vi "I2C_MASTER_READ.vi"(0 "error in (no error)":errorcluster) -> (1 "Arduino Data":T1, 2 "error out":errorcluster)   [LabVIEW 2018]
uses:
  <vilib>/Studica/Studica Toolkit/Background/I2C Channel.ctl
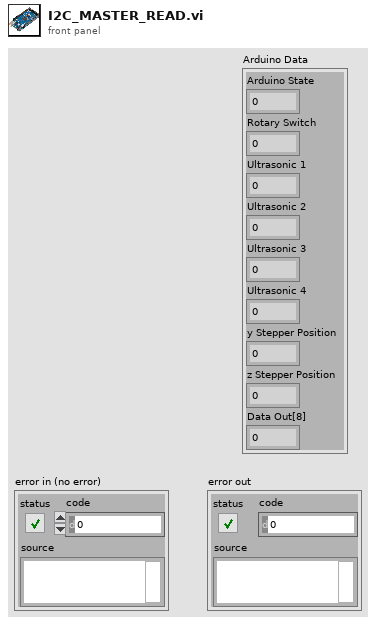
[diagram p1: front panel]
types:
  T1 = cluster{"Arduino State":u8, "Rotary Switch":u8, "Ultrasonic 1":u8, "Ultrasonic 2":u8, "Ultrasonic 3":u8, "Ultrasonic 4":u8, "y Stepper Position":u8, "z Stepper Position":u8, "Data Out[8]":u8}
  T2 = typedef "I2C Channel.ctl" = enum16{"Not Connected", "A", "B"}
  T3 = cluster{"I2C Channel":T2, "FPGA VI Reference Out":refnum<k20>}
  T4 = cluster{"Data Out[0]":u8, "Data Out[1]":u8, "Data Out[2]":u8, "Data Out[3]":u8, "Data Out[4]":u8, "Data Out[5]":u8, "Data Out[6]":u8, "Data Out[7]":u8, "Data Out[8]":u8}
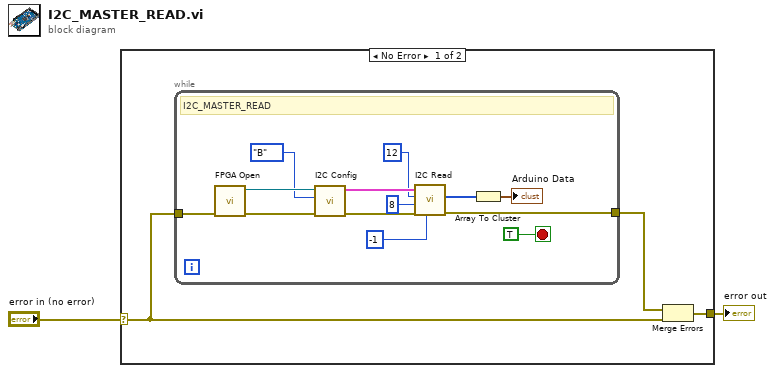
[diagram p0: block diagram]
diagram:
  n1 = case shown="No Error" "error in (no error)" {
    selector: "error in (no error)" -> [w3 w19]
    tunnel: [w5 w19] -> w1
    frame No Error {
      n2 = while {
        tunnel: [w7] -> w4
        tunnel: w3 -> [w6]
        stop <- TRUE stop-if-true
        # "I2C_MASTER_READ"
        n3 = call <vilib>:"FPGA Open.vi"("error in (no error)"=w6) -> ("error out"=w16:errorcluster, "FPGA Reference Out"=w18:refnum<k20>)  [unwired: 9 in]
        n4 = call <vilib>:"I2C Config.vi"("error in (no error)"=w16, "I2C Channel"=I2C_Channel."B", "FPGA Reference"=w18) -> ("error out"=w15:errorcluster, "I2C Ref Out"=w17:T3)  [unwired: 7 in]
        n5 = call <vilib>:"I2C Read.vi"("Timeout ms (1000)"=-1, "error in (no error)"=w15, "Bytes to Read"=u32 8, "Slave Address (7-bit)"=u8 12, "I2C Ref In"=w17) -> ("error out"=w7:errorcluster, "Data Out"=w13:u8[])  [unwired: 4 in, 1 out]
        n6 = Array To Cluster(array=w13) -> (cluster=→"Arduino Data":T4)
      }
      n7 = Merge Errors(w4, w3) -> (w5:errorcluster)
    }
    frame Error {
    }
  }
  "error out" <- w1
